vi "graph make.vi"(6 "Score_B":dbl, 9 "quarter_score_B":dbl[](array[numeric]), 10 "Score_A":dbl, 11 "quarter_score_A":dbl[](array[numeric])) -> (1 "Array 2":dbl[](array[numeric]), 2 "Array":dbl[][](array[numeric]), 3 "Array 3":dbl[](array[numeric]))   [LabVIEW 2021]
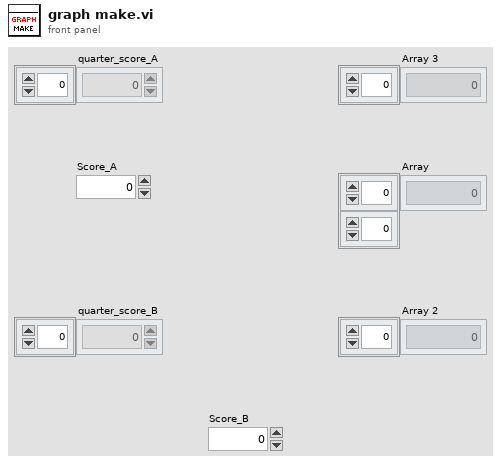
[diagram p1: front panel]
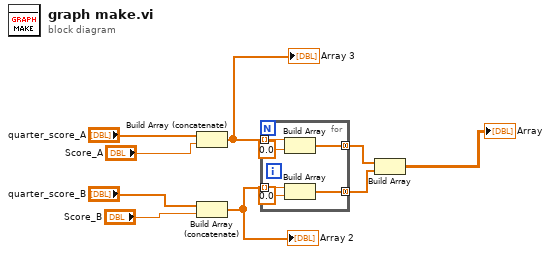
[diagram p0: block diagram]
diagram:
  n1 = Build Array (concatenate)("quarter_score_A", "Score_A") -> (w5:dbl[])
  "Array 3" <- w5
  n2 = Build Array (concatenate)("quarter_score_B", "Score_B") -> (w6:dbl[])
  "Array 2" <- w6
  n3 = for {
    tunnel: w5 -> [w15] mode=indexing
    tunnel: w6 -> [w12] mode=indexing
    tunnel: [w13] -> w8 mode=concatenating
    tunnel: [w10] -> w7 mode=concatenating
    n4 = Build Array(w15, 0.0 ("element")) -> (w13:dbl[])
    n5 = Build Array(w12, 0.0 ("element")) -> (w10:dbl[])
  }
  n6 = Build Array(w8, w7) -> (→"Array":dbl[][])
